vi "file write.vi"(1 "Array":dbl[](array[numeric]) format="%.2f", 2 "file path input":path) -> (0 "file path output":path)   [LabVIEW 2016]
uses:
  <vilib>/Utility/file.llb/Write To Spreadsheet File (DBL).vi
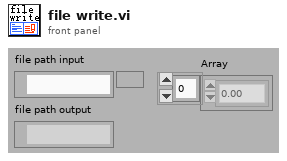
[diagram p1: front panel]
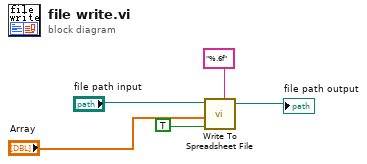
[diagram p0: block diagram]
diagram:
  n1 = call-poly <vilib>:"Write To Spreadsheet File.vi"("format (%.3f)"="%.6f", "append to file? (new file:F)"=TRUE, "1D data"="Array", "file path (dialog if empty)"="file path input") -> ("new file path (Not A Path if cancelled)"=→"file path output":path)  [unwired: 4 in]
